vi "Tools_String Match Wildcard Prefix.vi"(4 "case matching (sensitive)":T1=enum."system", 6 "offset (0)":i32, 7 "string":string, 8 "prefix with wildcards":string) -> (0 "offset past match":i32, 1 "found prefix":bool, 2 "after substring":string, 3 "match substring":string, 5 "before substring":string)   [LabVIEW 2017]
uses:
  Tools_String Case Matching.ctl
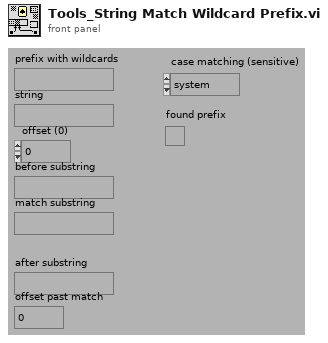
[diagram p1: front panel]
types:
  T1 = typedef "Tools_String Case Matching.ctl" = enum16{"a != A", "a == A", "system"}
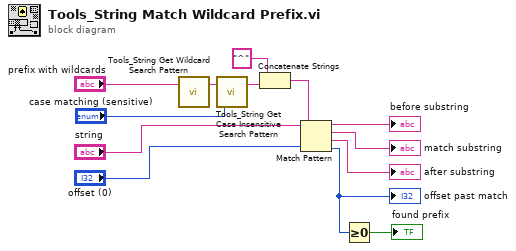
[diagram p0: block diagram]
diagram:
  n1 = call "Tools_String Get Wildcard Search Pattern.vi"("literal string"="prefix with wildcards") -> ("regular expression"=w7:string)  [unwired: 1 in, 1 out]
  n2 = call "Tools_String Get Case Insensitive Search Pattern.vi"("case matching (sensitive)"="case matching (sensitive)", "regular expression"=w7) -> ("case insensitive regular expression"=w3:string)  [unwired: 1 out]
  n3 = Concatenate Strings("^", w3) -> (w2:string)
  n4 = Match Pattern(string="string", regular expression=w2, offset (0)="offset (0)") -> (before substring=→"before substring":string, match substring=→"match substring":string, after substring=→"after substring":string, offset past match=w6:i32)
  "offset past match" <- w6
  n5 = Greater Or Equal To 0?(x=w6) -> (x >= 0?=→"found prefix":bool)
